vi "Fail if in Result.vi"(8 "error in (no error)":errorcluster, 9 "Results":T1[](array[typedef]), 10 "Method Name":string, 11 "LUnit Test Suite Tests in":refnum<class "LUnit Test Suite Tests.lvclass">) -> (0 "error out":errorcluster, 3 "LUnit Test Suite Tests out":refnum<class "LUnit Test Suite Tests.lvclass">)   [LabVIEW 2020, in "LUnit Test Suite Tests.lvclass"]
uses:
  LUnit Test Suite Tests.lvclass
  source/Core/Result/Result.ctl
  source/Core/Result/Status.ctl
  source/Core/Result/Type.ctl
  C:/Program Files (x86)/National Instruments/LabVIEW 2020/vi.lib/Astemes/LUnit/Test Case.lvclass
  <vilib>/Astemes/LUnit/Test Case.lvclass/Test Case.ctl
  <vilib>/Astemes/LUnit/Append Pass Result.vi
  <vilib>/Astemes/LUnit/Append Fail Result.vi
  <vilib>/Astemes/LUnit/Run In UI.vi
  <vilib>/Utility/error.llb/Clear Errors.vi
  <vilib>/Astemes/LUnit/Test Case.lvclass
  source/Core/Result/Result.lvlib
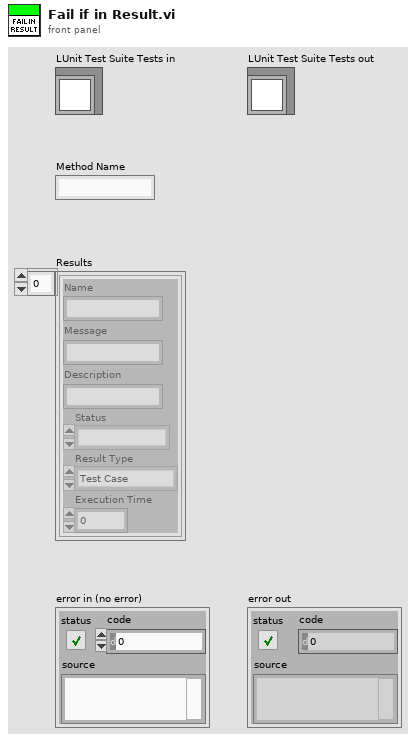
[diagram p1: front panel]
types:
  T1 = typedef "Result.lvlib/Result.ctl" = cluster{"Name":string, "Message":string, "Description":string, "Status":T2, "Result Type":T3, "Execution Time":dbl}
  T2 = typedef "Result.lvlib/Status.ctl" = enum16{"", "Passed", "Failed", "Error", "Skipped", "Setup Error", "Broken", "Teardown Error"}
  T3 = typedef "Result.lvlib/Type.ctl" = enum16{"Test Case", "Test Suite", "Test Run", "Pass", "Fail", "Skip", "Pass if", "Fail if", "Pass if Error", "Fail if Error", "Pass if Equal", "Fail if Equal"}
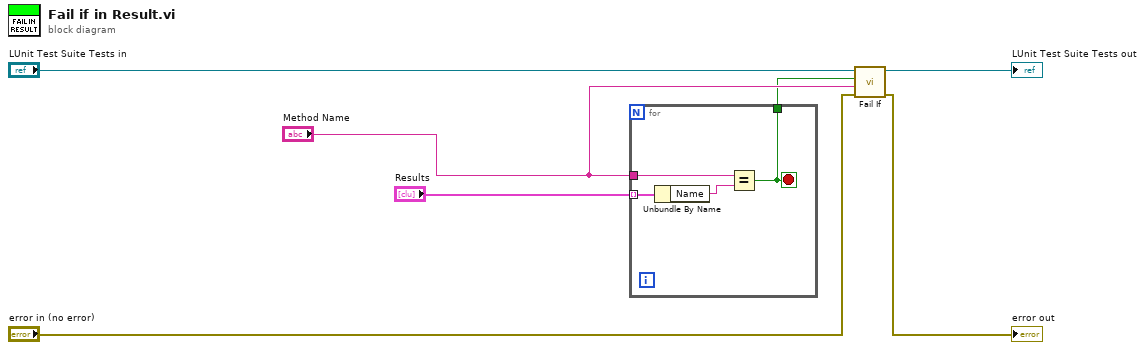
[diagram p0: block diagram]
diagram:
  n1 = for {
    tunnel: "Results" -> [w11] mode=indexing
    tunnel: "Method Name" -> [w9]
    tunnel: [w8] -> w6
    stop <- w8 stop-if-true
    n2 = Unbundle By Name(w11) -> ("Name"=w10:string)
    n3 = Equal?(x=w9, y=w10) -> (x = y?=w8:bool)
  }
  n4 = call <vilib>:"Fail If.vi"("error in (no error)"="error in (no error)", "Message"="Method Name", "Fail?"=w6, "LUnit Test Case In"="LUnit Test Suite Tests in") -> ("error out"=→"error out":errorcluster, "LUnit Test Case Out"=→"LUnit Test Suite Tests out":refnum<class "LUnit Test Suite Tests.lvclass">)  [unwired: 6 in]
